vi "PCO_RecorderSaveImage_B16.vi"(0 "pImgBuf":u16[][](array[numeric])=array1x4097[4097 elements], 1 "wWidth":u16, 2 "wHeight":u16, 3 "szFilePath":path, 5 "error in (no error)":errorcluster {"code" format="%x"}, 6 "isColor":bool, 8 "bIsBitmap":bool, 9 "PCO_METADATA_STRUCT":T1, 10 "bOverwrite":bool) -> (14 "ErrorMessage":i32 format="%x", 19 "error out":errorcluster {"code" format="%x"})   [LabVIEW 2019, in "Recorder.lvlib"]
doc: "int WINAPI PCO_RecorderSaveImage(void* pImgBuf, WORD wWidth, WORD wHeight, const char* cFileType, bool bIsBitmap, const char* szFilePath, bool bOverwrite, PCO_METADATA_STRUCT* strMetadata);"
uses:
  Recorder.lvlib
  pco.sdk/Structures/Structures.lvlib
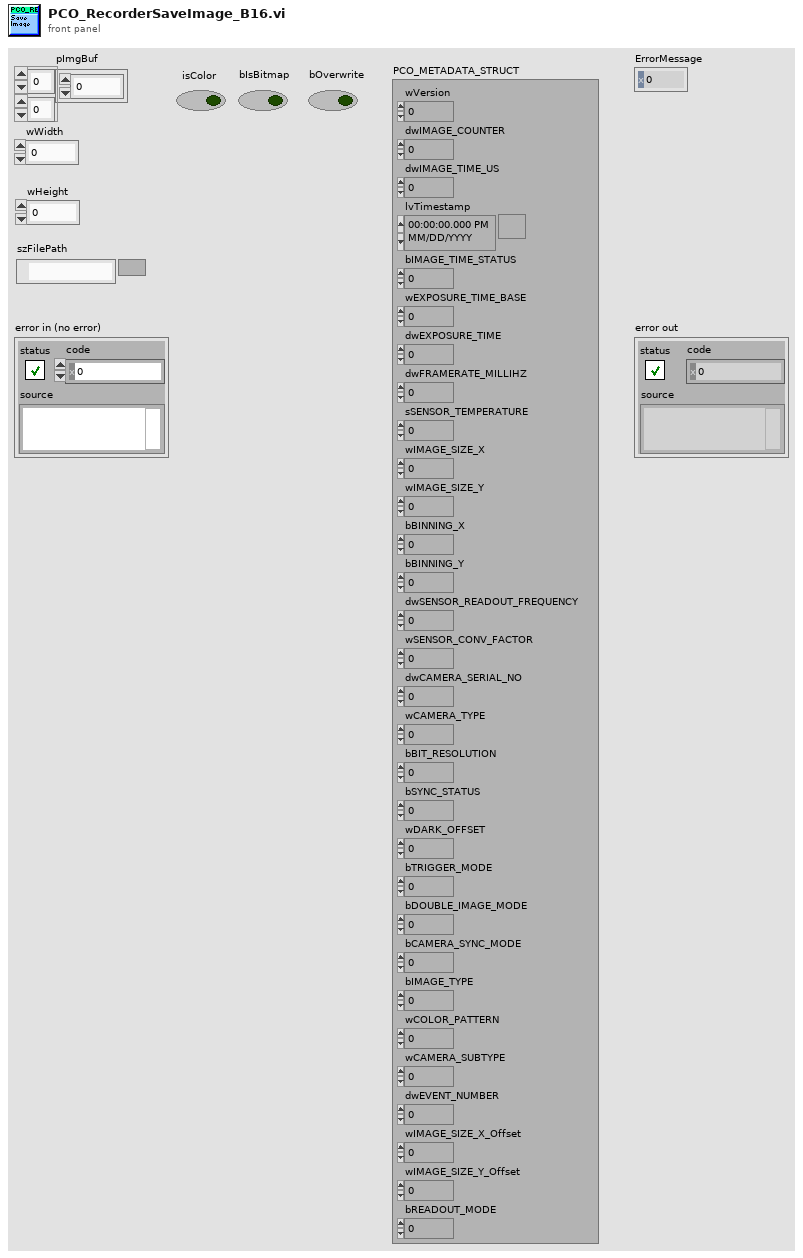
[diagram p1: front panel]
types:
  T1 = cluster{"wVersion":u16, "dwIMAGE_COUNTER":u32, "dwIMAGE_TIME_US":u32, "lvTimestamp":timestamp, "bIMAGE_TIME_STATUS":u8, "wEXPOSURE_TIME_BASE":u16, "dwEXPOSURE_TIME":u32, "dwFRAMERATE_MILLIHZ":u32, "sSENSOR_TEMPERATURE":i16, "wIMAGE_SIZE_X":u16, "wIMAGE_SIZE_Y":u16, "bBINNING_X":u8, "bBINNING_Y":u8, "dwSENSOR_READOUT_FREQUENCY":u32, "wSENSOR_CONV_FACTOR":u16, "dwCAMERA_SERIAL_NO":u32, "wCAMERA_TYPE":u16, "bBIT_RESOLUTION":u8, "bSYNC_STATUS":u8, "wDARK_OFFSET":u16, "bTRIGGER_MODE":u8, "bDOUBLE_IMAGE_MODE":u8, "bCAMERA_SYNC_MODE":u8, "bIMAGE_TYPE":u8, "wCOLOR_PATTERN":u16, "wCAMERA_SUBTYPE":u16, "dwEVENT_NUMBER":u32, "wIMAGE_SIZE_X_Offset":u16, "wIMAGE_SIZE_Y_Offset":u16, "bREADOUT_MODE":u8}
  T2 = typedef "LVDateTimeRec.ctl" = cluster{"fractional second":dbl, "second":i32, "minute":i32, "hour":i32, "day of month":i32, "month":i32, "year":i32, "day of week":i32, "day of year":i32, "DST":i32}
  T3 = cluster{"wSize":u16, "wVersion":u16, "bIMAGE_COUNTER_BCD":cluster{u8, u8, u8, u8}, "bIMAGE_TIME_US_BCD":cluster{u8, u8, u8}, "bIMAGE_TIME_SEC_BCD":u8, "bIMAGE_TIME_MIN_BCD":u8, "bIMAGE_TIME_HOUR_BCD":u8, "bIMAGE_TIME_DAY_BCD":u8, "bIMAGE_TIME_MON_BCD":u8, "bIMAGE_TIME_YEAR_BCD":u8, "bIMAGE_TIME_STATUS":u8, "wEXPOSURE_TIME_BASE":u16, "dwEXPOSURE_TIME":u32, "dwFRAMERATE_MILLIHZ":u32, "sSENSOR_TEMPERATURE":i16, "wIMAGE_SIZE_X":u16, "wIMAGE_SIZE_Y":u16, "bBINNING_X":u8, "bBINNING_Y":u8, "dwSENSOR_READOUT_FREQUENCY":u32, "wSENSOR_CONV_FACTOR":u16, "dwCAMERA_SERIAL_NO":u32, "wCAMERA_TYPE":u16, "bBIT_RESOLUTION":u8, "bSYNC_STATUS":u8, "wDARK_OFFSET":u16, "bTRIGGER_MODE":u8, "bDOUBLE_IMAGE_MODE":u8, "bCAMERA_SYNC_MODE":u8, "bIMAGE_TYPE":u8, "wCOLOR_PATTERN":u16, "wCAMERA_SUBTYPE":u16, "dwEVENT_NUMBER":u32, "wIMAGE_SIZE_X_Offset":u16, "wIMAGE_SIZE_Y_Offset":u16, "bREADOUT_MODE":u8}
  T4 = enum16{"big-endian, network order", "native, host order", "little-endian"}
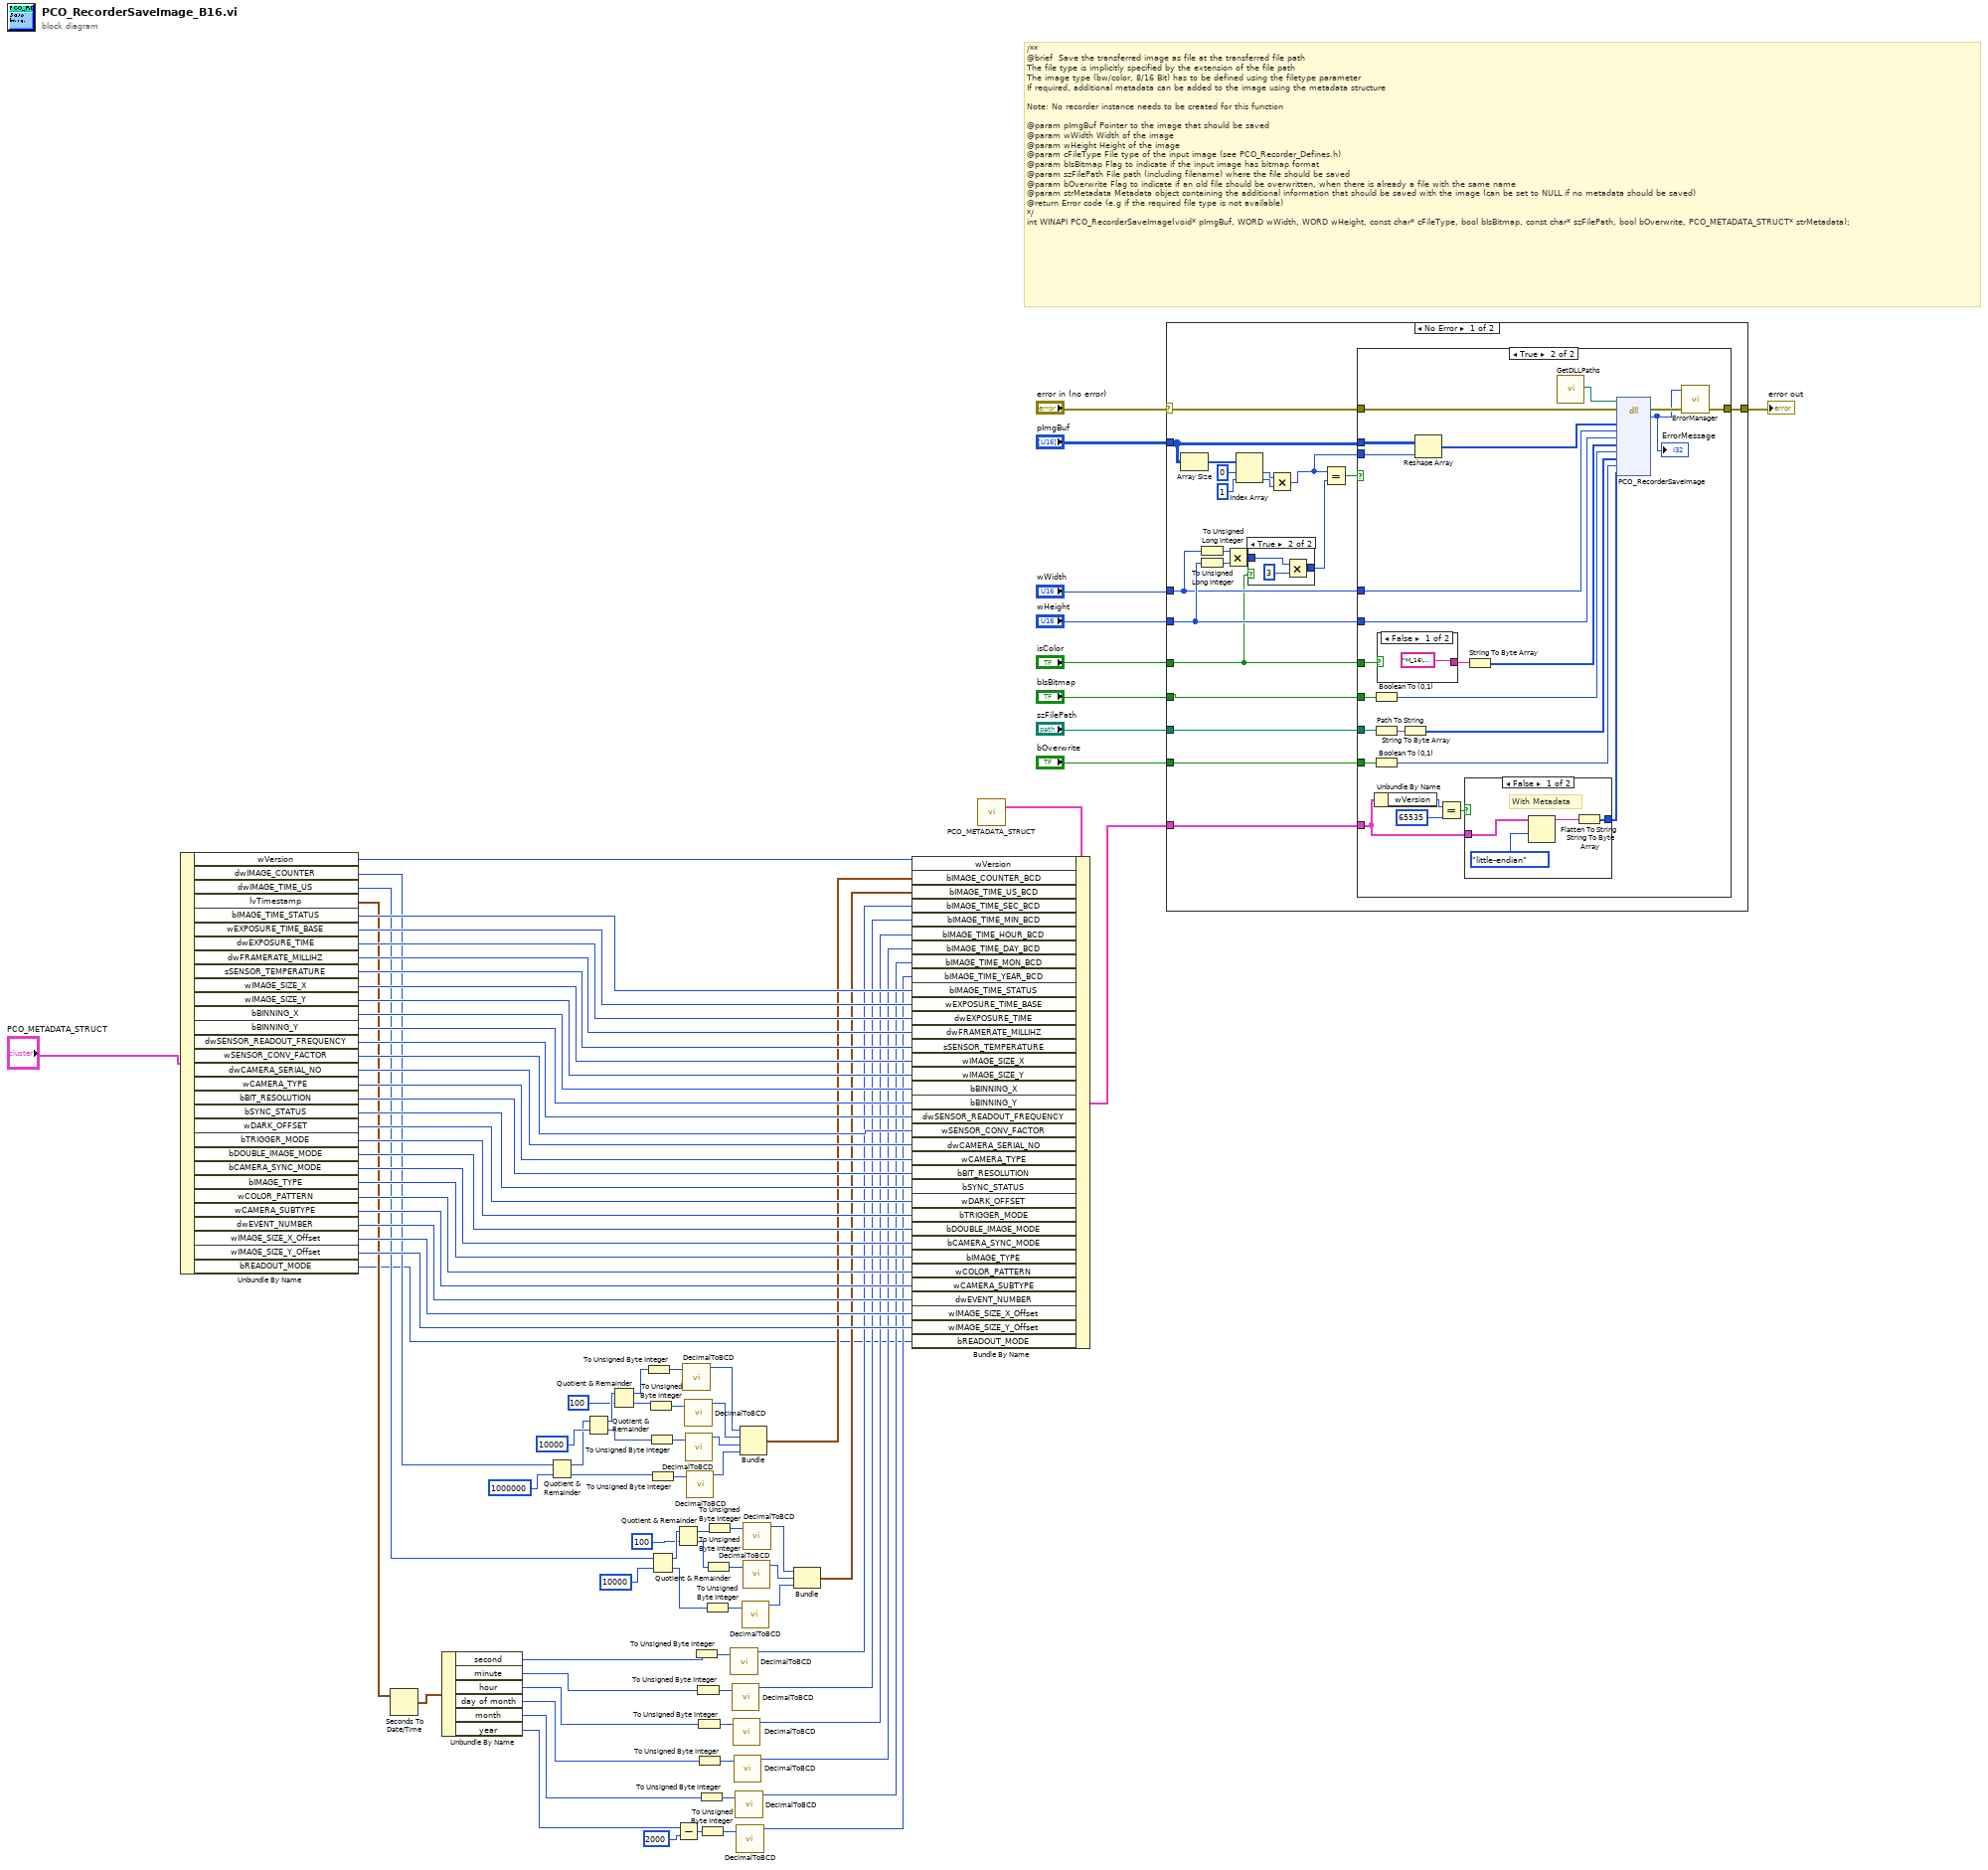
[diagram p0: block diagram]
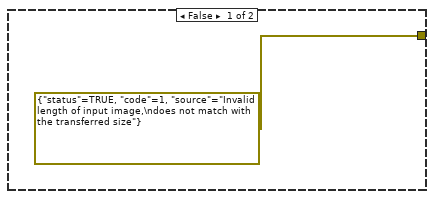
[diagram p3: hidden frame]
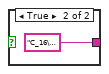
[diagram p4: hidden frame]
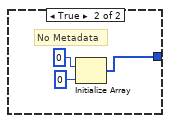
[diagram p5: hidden frame]
diagram:
  # "/**\n@brief  Save the transferred image as file at the transferred file path\nThe file type is implicitly specified by the extension of the file path\nThe image type (bw/color, 8/16 Bit) has to be defined using the filetype parameter\nIf required, additional metadata can be added to the image using the metadata structure\n\nNote: No recorder instance needs to be created for this function\n\n@param pImgBuf Pointer to the image that should be saved\n@param wWidth Width of the image\n@param wHeight Height of the image\n@param cFileType File type of the input image (see PCO_Recorder_Defines.h)\n@param bIsBitmap Flag to indicate if the input image has bitmap format\n@param szFilePath File path (including filename) where the file should be saved\n@param bOverwrite Flag to indicate if an old file should be overwritten, when there is already a file with the same name\n@param strMetadata Metadata object containing the additional information that should be saved with the image (can be set to NULL if no metadata should be saved)\n@return Error code (e.g if the required file type is not available)\n*/\nint WINAPI PCO_RecorderSaveImage(void* pImgBuf, WORD wWidth, WORD wHeight, const char* cFileType, bool bIsBitmap, const char* szFilePath, bool bOverwrite, PCO_METADATA_STRUCT* strMetadata);"
  n1 = Unbundle By Name("PCO_METADATA_STRUCT") -> ("wVersion"=w84:u16, "dwIMAGE_COUNTER"=w18:u32, "dwIMAGE_TIME_US"=w23:u32, "lvTimestamp"=w58:timestamp, "bIMAGE_TIME_STATUS"=w72:u8, "wEXPOSURE_TIME_BASE"=w59:u16, "dwEXPOSURE_TIME"=w60:u32, "dwFRAMERATE_MILLIHZ"=w61:u32, "sSENSOR_TEMPERATURE"=w62:i16, "wIMAGE_SIZE_X"=w63:u16, "wIMAGE_SIZE_Y"=w64:u16, "bBINNING_X"=w65:u8, "bBINNING_Y"=w66:u8, "dwSENSOR_READOUT_FREQUENCY"=w67:u32, "wSENSOR_CONV_FACTOR"=w68:u16, "dwCAMERA_SERIAL_NO"=w69:u32, "wCAMERA_TYPE"=w70:u16, "bBIT_RESOLUTION"=w71:u8, "bSYNC_STATUS"=w73:u8, "wDARK_OFFSET"=w74:u16, "bTRIGGER_MODE"=w75:u8, "bDOUBLE_IMAGE_MODE"=w76:u8, "bCAMERA_SYNC_MODE"=w77:u8, "bIMAGE_TYPE"=w78:u8, "wCOLOR_PATTERN"=w79:u16, "wCAMERA_SUBTYPE"=w80:u16, "dwEVENT_NUMBER"=w81:u32, "wIMAGE_SIZE_X_Offset"=w82:u16, "wIMAGE_SIZE_Y_Offset"=w83:u16, "bREADOUT_MODE"=w1:u8)
  n2 = Seconds To Date/Time(time stamp (now)=w58) -> (date time rec=w57:T2)  [unwired: 1 in]
  n3 = Unbundle By Name(w57) -> ("second"=w56:i32, "minute"=w53:i32, "hour"=w48:i32, "day of month"=w47:i32, "month"=w46:i32, "year"=w43:i32)
  n4 = Quotient & Remainder(x=w18, y=u32 1000000 ("x")) -> (x-y*floor(x/y)=w17:u32, floor(x/y)=w12:u32)
  n5 = Quotient & Remainder(x=w17, y=u32 10000 ("x")) -> (x-y*floor(x/y)=w21:u32, floor(x/y)=w11:u32)
  n6 = Quotient & Remainder(x=w21, y=u32 100 ("x")) -> (x-y*floor(x/y)=w9:u32, floor(x/y)=w10:u32)
  n7 = To Unsigned Byte Integer(number=w9) -> (unsigned 8bit integer=w16:u8)
  n8 = To Unsigned Byte Integer(number=w10) -> (unsigned 8bit integer=w15:u8)
  n9 = To Unsigned Byte Integer(number=w11) -> (unsigned 8bit integer=w14:u8)
  n10 = To Unsigned Byte Integer(number=w12) -> (unsigned 8bit integer=w13:u8)
  n11 = Quotient & Remainder(x=w23, y=u32 10000 ("x")) -> (x-y*floor(x/y)=w35:u32, floor(x/y)=w28:u32)
  n12 = Quotient & Remainder(x=w35, y=u32 100 ("x")) -> (x-y*floor(x/y)=w32:u32, floor(x/y)=w30:u32)
  n13 = Subtract(x=w43, y=2000) -> (x-y=w44:i32)
  n14 = call "DecimalToBCD.vi"("U8"=w16) -> ("BCD"=w8:u8)  [unwired: 10 in]
  n15 = call "DecimalToBCD.vi"("U8"=w15) -> ("BCD"=w7:u8)  [unwired: 10 in]
  n16 = call "DecimalToBCD.vi"("U8"=w14) -> ("BCD"=w6:u8)  [unwired: 10 in]
  n17 = call "DecimalToBCD.vi"("U8"=w13) -> ("BCD"=w5:u8)  [unwired: 10 in]
  n18 = To Unsigned Byte Integer(number=w56) -> (unsigned 8bit integer=w55:u8)
  n19 = To Unsigned Byte Integer(number=w53) -> (unsigned 8bit integer=w54:u8)
  n20 = To Unsigned Byte Integer(number=w48) -> (unsigned 8bit integer=w52:u8)
  n21 = To Unsigned Byte Integer(number=w47) -> (unsigned 8bit integer=w49:u8)
  n22 = To Unsigned Byte Integer(number=w46) -> (unsigned 8bit integer=w50:u8)
  n23 = To Unsigned Byte Integer(number=w44) -> (unsigned 8bit integer=w51:u8)
  n24 = To Unsigned Byte Integer(number=w28) -> (unsigned 8bit integer=w29:u8)
  n25 = To Unsigned Byte Integer(number=w30) -> (unsigned 8bit integer=w31:u8)
  n26 = To Unsigned Byte Integer(number=w32) -> (unsigned 8bit integer=w33:u8)
  n27 = call "DecimalToBCD.vi"("U8"=w55) -> ("BCD"=w37:u8)  [unwired: 10 in]
  n28 = call "DecimalToBCD.vi"("U8"=w54) -> ("BCD"=w38:u8)  [unwired: 10 in]
  n29 = call "DecimalToBCD.vi"("U8"=w52) -> ("BCD"=w39:u8)  [unwired: 10 in]
  n30 = call "DecimalToBCD.vi"("U8"=w49) -> ("BCD"=w40:u8)  [unwired: 10 in]
  n31 = call "DecimalToBCD.vi"("U8"=w50) -> ("BCD"=w41:u8)  [unwired: 10 in]
  n32 = call "DecimalToBCD.vi"("U8"=w51) -> ("BCD"=w42:u8)  [unwired: 10 in]
  n33 = Bundle("BCD"=w8, "BCD"=w7, "BCD"=w6, "BCD"=w5) -> (w4:cluster{"BCD":u8, "BCD":u8, "BCD":u8, "BCD":u8})  [unwired: 1 in]
  n34 = call "DecimalToBCD.vi"("U8"=w29) -> ("BCD"=w25:u8)  [unwired: 10 in]
  n35 = call "DecimalToBCD.vi"("U8"=w31) -> ("BCD"=w26:u8)  [unwired: 10 in]
  n36 = call "DecimalToBCD.vi"("U8"=w33) -> ("BCD"=w27:u8)  [unwired: 10 in]
  n37 = Bundle("BCD"=w27, "BCD"=w26, "BCD"=w25) -> (w24:cluster{"BCD":u8, "BCD":u8, "BCD":u8})  [unwired: 1 in]
  n38 = call "PCO_METADATA_STRUCT.vi"() -> ("PCO_METADATA_STRUCT_Raw"=w85:T3)  [unwired: 4 in, 3 out]
  n39 = Bundle By Name(cluster=w85, "wVersion"=w84, "bIMAGE_COUNTER_BCD"=w4, "bIMAGE_TIME_US_BCD"=w24, "bIMAGE_TIME_SEC_BCD"=w37, "bIMAGE_TIME_MIN_BCD"=w38, "bIMAGE_TIME_HOUR_BCD"=w39, "bIMAGE_TIME_DAY_BCD"=w40, "bIMAGE_TIME_MON_BCD"=w41, "bIMAGE_TIME_YEAR_BCD"=w42, "bIMAGE_TIME_STATUS"=w72, "wEXPOSURE_TIME_BASE"=w59, "dwEXPOSURE_TIME"=w60, "dwFRAMERATE_MILLIHZ"=w61, "sSENSOR_TEMPERATURE"=w62, "wIMAGE_SIZE_X"=w63, "wIMAGE_SIZE_Y"=w64, "bBINNING_X"=w65, "bBINNING_Y"=w66, "dwSENSOR_READOUT_FREQUENCY"=w67, "wSENSOR_CONV_FACTOR"=w68, "dwCAMERA_SERIAL_NO"=w69, "wCAMERA_TYPE"=w70, "bBIT_RESOLUTION"=w71, "bSYNC_STATUS"=w73, "wDARK_OFFSET"=w74, "bTRIGGER_MODE"=w75, "bDOUBLE_IMAGE_MODE"=w76, "bCAMERA_SYNC_MODE"=w77, "bIMAGE_TYPE"=w78, "wCOLOR_PATTERN"=w79, "wCAMERA_SUBTYPE"=w80, "dwEVENT_NUMBER"=w81, "wIMAGE_SIZE_X_Offset"=w82, "wIMAGE_SIZE_Y_Offset"=w83, "bREADOUT_MODE"=w1) -> (w3:T3)
  n40 = case shown="No Error" "error in (no error)" {
    selector: "error in (no error)" -> [w114 w155]
    tunnel: "pImgBuf" -> [w113 _]
    tunnel: "wWidth" -> [w96 _]
    tunnel: "wHeight" -> [w97 _]
    tunnel: "bIsBitmap" -> [w107 _]
    tunnel: [w115 w155] -> w90
    tunnel: "szFilePath" -> [w108 _]
    tunnel: "bOverwrite" -> [w109 _]
    tunnel: "isColor" -> [w95 _]
    tunnel: w3 -> [w110 _]
    frame No Error {
      n41 = Array Size(array=w113) -> (size(s)=w106:i32[])
      n42 = To Unsigned Long Integer(number=w96) -> (unsigned 32bit integer=w99:u32)
      n43 = To Unsigned Long Integer(number=w97) -> (unsigned 32bit integer=w98:u32)
      n44 = Multiply(x=w99, y=w98) -> (x*y=w112:u32)
      n45 = Index Array(array=w106, index #1=0 ("index"), index #2=1 ("index")) -> (element #1=w104:i32, element #2=w102:i32)
      n46 = case shown="True" w95 {
        tunnel: w112 -> [w116 w119]
        tunnel: [w116 w117] -> w101
        frame False {
        }
        frame True {
          n47 = Multiply(x=w119, y=u16 3) -> (x*y=w117:u32)
        }
      }
      n48 = Multiply(x=w104, y=w102) -> (x*y=w100:i32)
      n49 = Equal?(x=w100, y=w101) -> (x = y?=w111:bool)
      n50 = case shown="True" w111 {
        tunnel: w113 -> [_ w123]
        tunnel: w96 -> [_ w145]
        tunnel: w97 -> [_ w144]
        tunnel: w107 -> [_ w143]
        tunnel: [errorcluster {"status"=TRUE, "code"=1, "source"="Invalid length of input image,\ndoes not match with the transferred size"} ("error out") w137] -> w115
        tunnel: w114 -> [_ w140]
        tunnel: w95 -> [_ w129]
        tunnel: w110 -> [_ w131]
        tunnel: w109 -> [_ w130]
        tunnel: w108 -> [_ w127]
        tunnel: w100 -> [_ w121]
        frame False {
        }
        frame True {
          n51 = Boolean To (0,1)(Boolean=w143) -> (0, 1=w142:i16)
          n52 = Path To String(path=w127) -> (string=w128:string)
          n53 = Boolean To (0,1)(Boolean=w130) -> (0, 1=w141:i16)
          n54 = Unbundle By Name(w131) -> ("wVersion"=w135:u16)
          n55 = case shown="False" w129 {
            tunnel: ["M_16\u0000" "C_16\u0000"] -> w125
            frame False {
            }
            frame True {
            }
          }
          n56 = String To Byte Array(string=w128) -> (unsigned byte array=w126:u8[])
          n57 = Reshape Array(w123, w121) -> (w122:u16[])
          n58 = Equal?(x=w135, y=u16 65535) -> (x = y?=w133:bool)
          n59 = case shown="False" w133 {
            tunnel: [w149 w152] -> w132
            tunnel: w131 -> [w150 _]
            frame False {
              # "With Metadata"
              n60 = Flatten To String(anything=w150, byte order (0:big-endian, network order)=T4."little-endian" ("Byte-Reihenfolge (0:Big-Endian, Netzwerkreihenfolge)")) -> (data string=w151:string)  [unwired: 2 in, 2 out]
              n61 = String To Byte Array(string=w151) -> (unsigned byte array=w149:u8[])
            }
            frame True {
              # "No Metadata"
              n62 = Initialize Array(u8 0, 0 ("dimension size")) -> (w152:u8[])
            }
          }
          n63 = String To Byte Array(string=w125) -> (unsigned byte array=w124:u8[])
          n64 = call "GetDLLPaths.vi"() -> ("PCO_Recorder_Path"=w139:path)  [unwired: 8 in, 3 out]
          n65 = dll-call lib="?" fn="PCO_RecorderSaveImage"(path in=w139, error in=w140, "pImgBuf"=w122, "wWidth"=w145, "wHeight"=w144, "cFileType"=w124, "bIsBitmap"=w142, "szFilePath"=w126, "bOverwrite"=w141, "strMetadata"=w132) -> (error out=w138:errorcluster, "return type"=w136:i32)  [unwired: 9 in, 1 out]
          "ErrorMessage" <- w136
          n66 = call "ErrorManager.vi"("error in (no error)"=w138, "error code"=w136) -> ("error out"=w137:errorcluster)  [unwired: 2 in, 1 out]
        }
      }
    }
    frame Error {
    }
  }
  "error out" <- w90
